vi "CRYResonance Nonlinear Lev-Mar Fit.vi"(5 "derivative":T1(ring), 6 "Standard Deviation":dbl[](array[numeric]) format="%.2f", 7 "max iteration":i32=5000, 8 "Initial Guess Coefficients":dbl[](array[numeric])=[1.776184495703007e-07, -0.14085158207570353, 40088.565947040355] format="%.2e", 9 "Y":dbl[](array[numeric])=[3.9898896139061897, 4.3124733116327585, 4.876614663326357, 5.3456167821063225, 5.780646113329947, 5.931389362641254, 5.945906297373114, 5.824185536388709, 5.319519758494435, 4.994682380787082, 4.41488466631378, 3.9582428120619126, 3.655735938066415] format="%.2f", 10 "X":dbl[](array[numeric])=[79.62143411069965, 84.33930068571668, 89.33671843019287, 94.63025179229638, 100.23744672545476, 106.176888846198, 112.46826503807017, 119.13242870580248, 126.19146889603907, 133.66878351372338, 141.58915687682807, 149.97884186649168, 158.86564694485688] format="%.2f") -> (0 "error":i32=-20041, 1 "mse":dbl=nan format="%.4e", 2 "Best Fit":dbl[](array[numeric]) format="%.2f", 3 "Best Fit Coefficients":dbl[](array[numeric]) format="%.2e", 4 "Covariance":dbl[][](array[numeric]) format="%.2f")   [LabVIEW 2013]
doc: "NonLinear Lev-Mar Fit:\n==================\n\nThis VI uses the Levenberg-Marquardt algorithm to determine the least squares set of coefficients that best fit the set of input data points(X,Y) as expressed by a nonlinear function y=f(x,a) where a is the set of coefficients. This VI also gives the best fit curve y=f(x.a). \n\nThe user needs to open a sub-VI \"Target Fnc & Deriv NonLin\" and inputs his/her nonlinear function f(x,a) in the Formula Node. If the user choose formula caculation for derivative method, he/she needs to input the partial deriative of f(x,a) with respect to a as well. \n\nInputs:\nX: experiment data points.\nY: experiment data points.\nStandard Deviation: standard deviation of each experiment data.If you don't have knowledge about this parameter, just leave it empty.\nInitial Guess Coefficients: Your guessed coefficients. If this is too far from the appropriate coefficients, the VI maybe will fail to return the appropriate coeficients and best fit curve.\nmax iteration: max iteration the algrothim will try. If it can not converge when it reaches the max iteration. The VI will return an error.\nderivative: There are two ways to caculate the partial derivative of f(x,a) with respect to coefficients a. If you choose nemerical caculation, the VI will use numerical method to caculate them internally. If you choose formula caculation, you need to input the derivative formula in the subvi Target Fnc & Deriv NonLin. formula caculation is more precise than numerical caculation.\n\nOutputs:\nBest Guess Coefficients: the least squares coefficients.\nBest Fit: the best fit curve f(x,a).\nCovariance: covariance matrix of Best Guess Coefficients.\nmse: mse=1/n*sum[(y(i)-f(x(i),a))/std(i)]^2)\n (std: Standard Deviation)"
uses:
  <vilib>/Analysis/baseanly.llb/Real Inverse Matrix.vi
  <vilib>/Analysis/NI_AALPro.lvlib
  <vilib>/Analysis/NI_AALBase.lvlib
panel:
  # "Nonlinear  Lev-Mar  Fit"
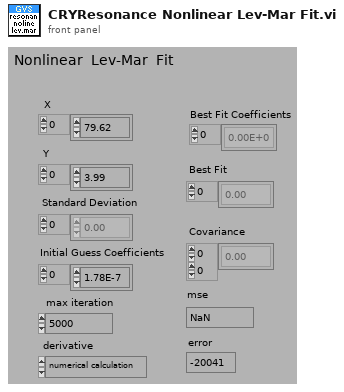
[diagram p1: front panel]
types:
  T1 = enum32{"numerical calculation", "formula calculation"}
  T2 = typedef "NI_Matrix.lvlib/RealMatrix.ctl" = dbl[][]
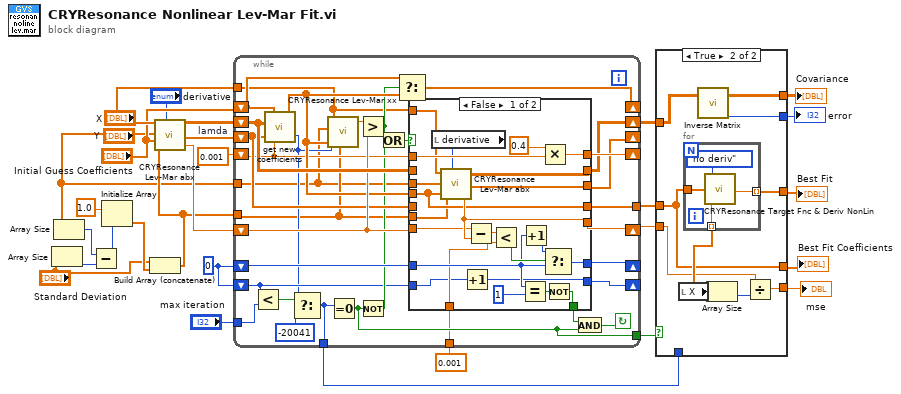
[diagram p0: block diagram]
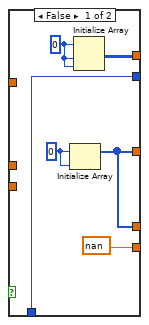
[diagram p2: hidden frame]
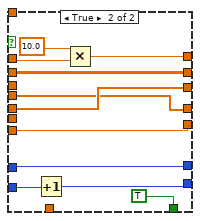
[diagram p3: hidden frame]
diagram:
  w17 = 0
  w26 = 0.001  # lamda
  n1 = Array Size(array="Standard Deviation") -> (size(s)=w6:i32)
  n2 = Array Size(array="Y") -> (size(s)=w7:i32)
  n3 = Subtract(x=w7, y=w6) -> (x-y=w5:i32)
  n4 = Initialize Array(1.0, w5) -> (w4:dbl[])
  n5 = Build Array (concatenate)("Standard Deviation", w4) -> (w2:dbl[])
  n6 = call "CRYResonance Lev-Mar abx.vi"("X"="X", "Y"="Y", "Coefficients"="Initial Guess Coefficients", "Standard Deviation"=w2, "derivative"="derivative") -> ("Alpha"=w27:dbl[][], "Beta"=w25:dbl[], "chiSqr"=w24:dbl)
  n7 = while {
    shift-right: [w59] -> _
    shift-left: w26 -> [w48]
    shift-right: [w58] -> _
    shift-left: "Initial Guess Coefficients" -> [w30]
    shift-right: [w57] -> w8
    shift-left: w27 -> [w56]
    shift-right: [w55] -> _
    shift-left: w25 -> [w50]
    shift-right: [w54] -> w23
    shift-left: w24 -> [w53]
    shift-right: [w51] -> _
    shift-left: w17 -> [w52]
    tunnel: [w47] -> w22
    tunnel: [w44] -> w19
    tunnel: 0.001 -> [w43]
    shift-right: [w39] -> _
    shift-left: w17 -> [w38]
    tunnel: w2 -> [w33]
    tunnel: "max iteration" -> [w34]
    tunnel: [w32] -> w9
    tunnel: "Y" -> [w31]
    tunnel: "X" -> [w29]
    stop <- w46 continue-if-true
    n8 = Less?(x=w38, y=w34) -> (x < y?=w37:bool)
    n9 = call <vilib>:"get new coefficients.vi"("lamda"=w48, "Beta"=w50, "Alpha"=w56, "Coefficients"=w30) -> ("error"=w35:i32, "New Coefficients"=w49:dbl[])
    n10 = Select(t=w35, s=w37, f=-20041) -> (s? t:f=w32:i32)
    n11 = call "CRYResonance Lev-Mar xx.vi"("X"=w29, "Y"=w31, "Coefficients"=w49, "error"=w35, "Standard Deviation"=w33) -> ("chiSqr"=w60:dbl)
    n12 = Equal To 0?(x=w32) -> (x = 0?=w44:bool)
    n13 = Greater?(x=w60, y=w53) -> (0:w41:bool)
    n14 = Not(x=w44) -> (.not. x?=w40:bool)
    n15 = Or(x=w41, y=w40) -> (x .or. y?=w42:bool)
    n16 = Select(t=w30, s=w41, f=w49) -> (s? t:f=w58:dbl[])
    n17 = case shown="False" w42 {
      tunnel: w48 -> [w82 w93]
      tunnel: [w81 w92] -> w59
      tunnel: [w80 w91] -> w57
      tunnel: w56 -> [_ w91]
      tunnel: [w79 w87] -> w55
      tunnel: [w78 w90] -> w54
      tunnel: w53 -> [w77 w90]
      tunnel: w52 -> [w72 w89]
      tunnel: [w73 w89] -> w51
      tunnel: [w69 TRUE] -> w45
      tunnel: w49 -> [w66 w86]
      tunnel: w50 -> [_ w87]
      tunnel: [w66 w86] -> w47
      tunnel: w43 -> [w68 _]
      tunnel: [w63 w85] -> w39
      tunnel: w38 -> [w67 w84]
      tunnel: w33 -> [w65 _]
      tunnel: w29 -> [w62 _]
      tunnel: w31 -> [w61 _]
      frame False {
        n18 = local read "derivative"() -> (w64:T1)
        n19 = call "CRYResonance Lev-Mar abx.vi"("X"=w62, "Y"=w61, "Coefficients"=w66, "Standard Deviation"=w65, "derivative"=w64) -> ("Alpha"=w80:dbl[][], "Beta"=w79:dbl[], "chiSqr"=w78:dbl)
        n20 = Increment(x=w67) -> (x+1=w63:i32)
        n21 = Subtract(x=w77, y=w78) -> (x-y=w76:dbl)
        n22 = Less?(x=w76, y=w68) -> (x < y?=w75:bool)
        n23 = Equal?(x=w72, y=1) -> (x = y?=w70:bool)
        n24 = Increment(x=w72) -> (x+1=w74:i32)
        n25 = Multiply(x=0.4, y=w82) -> (x*y=w81:dbl)
        n26 = Select(t=w74, s=w75, f=w72) -> (s? t:f=w73:i32)
        n27 = Not(x=w70) -> (.not. x?=w69:bool)
      }
      frame True {
        n28 = Increment(x=w84) -> (x+1=w85:i32)
        n29 = Multiply(x=10.0, y=w93) -> (x*y=w92:dbl)
      }
    }
    n30 = And(x=w45, y=w44) -> (x .and. y?=w46:bool)
  }
  n31 = case shown="True" w19 {
    tunnel: w22 -> [_ w105]
    tunnel: [w98 w105] -> w21
    tunnel: [nan w109] -> w20
    tunnel: [w98 w106] -> w12
    tunnel: w23 -> [_ w104]
    tunnel: [w96 w103] -> w11
    tunnel: [w95 w102] -> w10
    tunnel: w9 -> [w95 _]
    tunnel: w8 -> [_ w101]
    frame False {
      w97 = 0
      w100 = 0
      n32 = Initialize Array(w100, w100) -> (w98:i32[])
      n33 = Initialize Array(w97, w97, w97) -> (w96:i32[][])
    }
    frame True {
      n34 = local read "X"() -> (w108:dbl[])
      n35 = for {
        tunnel: w105 -> [w112]
        tunnel: [w111] -> w106 mode=indexing
        tunnel: w108 -> [w113] mode=indexing
        n36 = call "CRYResonance Target Fnc & Deriv NonLin.vi"("X"=w113, "Coefficients"=w112, "Flag"=enum16{"no deriv", "deriv"}."no deriv") -> ("Y"=w111:dbl)  [unwired: 1 out]
      }
      n37 = call-poly <vilib>:"Inverse Matrix.vi"("Input Matrix"=w101) -> ("error"=w102:i32, "Inverse Matrix"=w103:T2)  [unwired: 1 in]
      n38 = Array Size(array=w108) -> (size(s)=w107:i32)
      n39 = Divide(x=w104, y=w107) -> (x/y=w109:dbl)
    }
  }
  "mse" <- w20
  "Best Fit Coefficients" <- w21
  "Best Fit" <- w12
  "error" <- w10
  "Covariance" <- w11
